vi "Decimate DFD (Fs).vi"(6 "Nyquist Filter [F]":bool, 8 "error in (no error)":errorcluster, 9 "output fs (Hz)":dbl=6500.0 format="%#_13g", 10 "Fs":dbl, 11 "Waveforms in":waveform(dbl)[](array[waveform])) -> (0 "error out":errorcluster, 3 "waveforms out":waveform(dbl)[](array[waveform]))   [LabVIEW 2019, in "DSP.lvclass"]
uses:
  DSP.lvclass
  Decimate DFD (Array).vi/949379ad-8373-41eb-be01-93a6c1c1afb3.vi
  Decimate DFD (Array).vi/efb08f77-0c38-4651-8a9c-351b9595fc15.vi
panel:
  out "Decimation Factor":i32
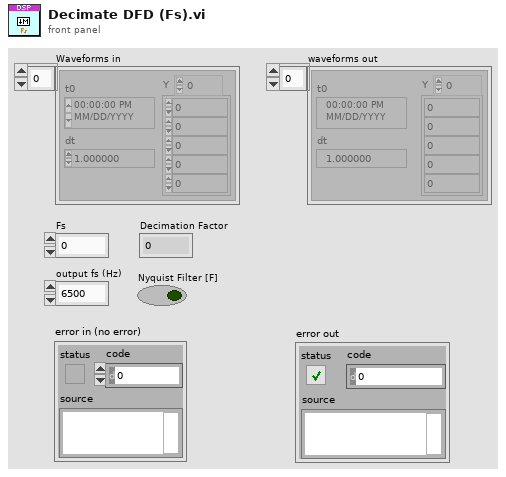
[diagram p1: front panel]
types:
  T1 = cluster{"filter structure":enum32{"IIR 2nd Order", "IIR 4th Order"}, "Reverse Coefficients":dbl[], "Forward Coefficients":dbl[]}[]
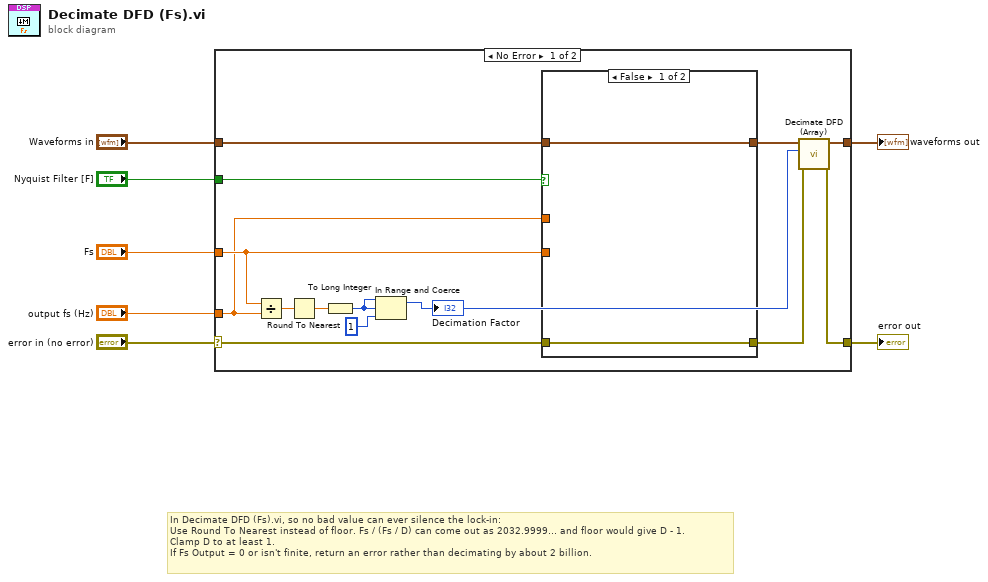
[diagram p0: block diagram]
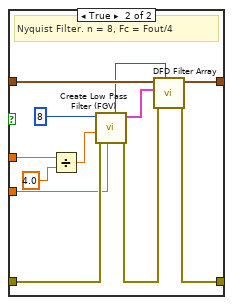
[diagram p2: hidden frame]
diagram:
  # "In Decimate DFD (Fs).vi, so no bad value can ever silence the lock-in:\nUse Round To Nearest instead of floor. Fs / (Fs / D) can come out as 2032.9999… and floor would give D - 1.\nClamp D to at least 1.\nIf Fs Output = 0 or isn't finite, return an error rather than decimating by about 2 billion."
  n1 = case shown="No Error" "error in (no error)" {
    selector: "error in (no error)" -> [w16 w37]
    tunnel: "output fs (Hz)" -> [w13 _]
    tunnel: "Waveforms in" -> [w17 w36]
    tunnel: [w19 w37] -> w4
    tunnel: [w20 w36] -> w3
    tunnel: "Fs" -> [w14 _]
    tunnel: "Nyquist Filter [F]" -> [w12 _]
    frame No Error {
      n2 = Divide(x=w14, y=w13) -> (x/y=w21:dbl)
      n3 = Round To Nearest(number=w21) -> (nearest integer value=w11:dbl)
      n4 = To Long Integer(number=w11) -> (32bit integer=w8:i32)
      n5 = In Range and Coerce(upper limit=w8, x=w8, lower limit=1) -> (coerced(x)=w10:i32)  [unwired: 1 out]
      "Decimation Factor" <- w10
      n6 = case shown="False" w12 {
        tunnel: [w23 w35] -> w18
        tunnel: w17 -> [w23 w34]
        tunnel: w16 -> [w22 w32]
        tunnel: [w22 w30] -> w15
        tunnel: w14 -> [_ w27]
        tunnel: w13 -> [_ w26]
        frame False {
        }
        frame True {
          # "Nyquist Filter. n = 8, Fc = Fout/4"
          n7 = Divide(x=w26, y=4.0) -> (x/y=w24:dbl)
          n8 = call "Create Low Pass Filter (FGV).vi"("fs (Hz)"=w27, "error in (no error)"=w32, "Low Pass Cutoff (Hz)"=w24, "order"=8) -> ("error out"=w31:errorcluster, "IIR Filters"=w28:T1, "init out"=w33:bool)  [unwired: 5 in]
          n9 = call "DFD Filter Array.vi"("init (F)"=w33, "error in (no error)"=w31, "IIR Filters"=w28, "signal in"=w34) -> ("error out"=w30:errorcluster, "signal out"=w35:waveform(dbl)[])  [unwired: 6 in]
        }
      }
      n10 = call "Decimate DFD (Array).vi"("error in (no error)"=w15, "Decimation Factor"=w10, "Waveforms in"=w18) -> ("error out"=w19:errorcluster, "waveforms out"=w20:waveform(dbl)[])  [unwired: 7 in]
    }
    frame Error {
    }
  }
  "waveforms out" <- w3
  "error out" <- w4
